vi "calculate_frequency_params.vi"(2 "Frequency 2":dbl, 3 "Frequency 1":dbl, 4 "Position 2":dbl, 5 "Position 1":dbl) -> (0 "Intercept":dbl, 1 "Slope":dbl)   [LabVIEW 2010]
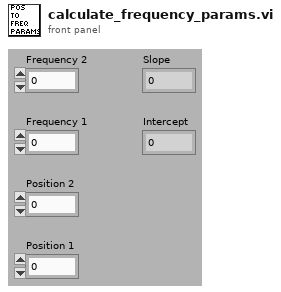
[diagram p1: front panel]
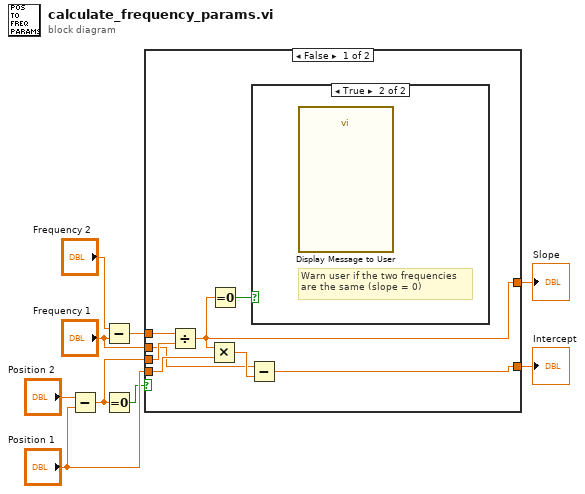
[diagram p0: block diagram]
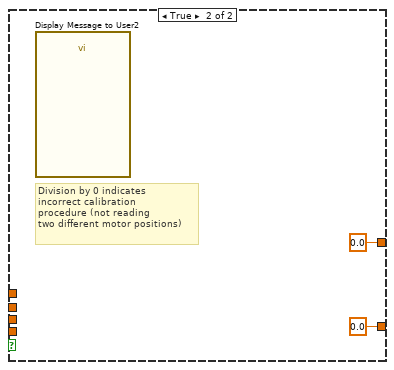
[diagram p3: hidden frame]
diagram:
  n1 = Subtract(x="Position 2", y="Position 1") -> (x-y=w4:dbl)
  n2 = Subtract(x="Frequency 2", y="Frequency 1") -> (x-y=w5:dbl)
  n3 = Equal To 0?(x=w4) -> (x = 0?=w3:bool)
  n4 = case shown="False" w3 {
    tunnel: w4 -> [w17 _]
    tunnel: w5 -> [w16 _]
    tunnel: "Position 1" -> [w15 _]
    tunnel: "Frequency 1" -> [w13 _]
    tunnel: [w10 0.0] -> w8
    tunnel: [w11 0.0] -> w9
    frame False {
      n5 = Divide(x=w16, y=w17) -> (x/y=w10:dbl)
      n6 = Multiply(x=w10, y=w15) -> (x*y=w14:dbl)
      n7 = Equal To 0?(x=w10) -> (x = 0?=w12:bool)
      n8 = Subtract(x=w13, y=w14) -> (x-y=w11:dbl)
      n9 = case shown="True" w12 {
        frame False {
        }
        frame True {
          # "Warn user if the two frequencies\nare the same (slope = 0)"
          n10 = call "Display Message to User"() -> ()  [unwired: 10 in, 2 out]
        }
      }
    }
    frame True {
      # "Division by 0 indicates\nincorrect calibration\nprocedure (not reading\ntwo different motor positions)"
      n11 = call "Display Message to User2"() -> ()  [unwired: 10 in, 2 out]
    }
  }
  "Intercept" <- w9
  "Slope" <- w8
